vi "Read Data.vi"(8 "error in":errorcluster, 11 "Waveform Data in":refnum<class "Waveform Data.lvclass">) -> (0 "error out":errorcluster, 2 "Data":waveform(dbl), 3 "Waveform Data out":refnum<class "Waveform Data.lvclass">)   [LabVIEW 2014, in "Base Data Class.lvlib" / "Waveform Data.lvclass"]
uses:
  Waveform Data.lvclass
  Waveform Data.lvclass/Waveform Data.ctl
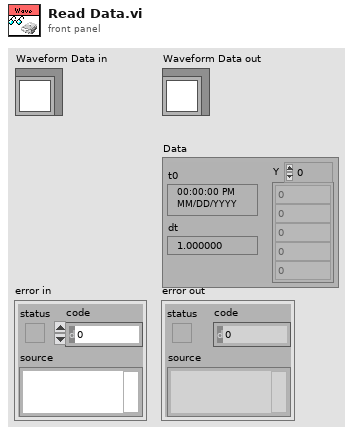
[diagram p1: front panel]
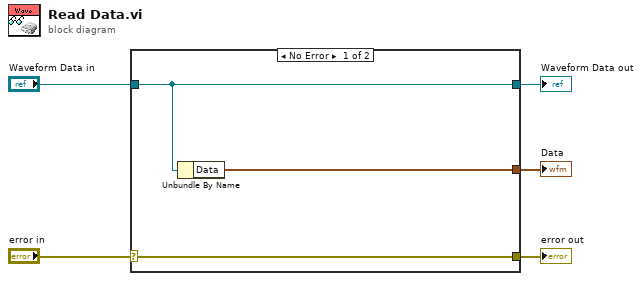
[diagram p0: block diagram]
diagram:
  n1 = case shown="No Error" "error in" {
    selector: "error in" -> [w8 w9]
    tunnel: [w8 w9] -> w4
    tunnel: [w7 w10] -> w2
    tunnel: "Waveform Data in" -> [w7 w10]
    tunnel: [w6 _] -> w1
    frame No Error {
      n2 = Unbundle By Name(w7) -> ("Data"=w6:waveform(dbl))
    }
    frame Error {
    }
  }
  "error out" <- w4
  "Waveform Data out" <- w2
  "Data" <- w1
